vi "get supported types.vi"(8 "error in":errorcluster, 11 "EthernetIP configuration in":refnum<class "EIP Tags Configuration.lvclass">) -> (0 "error out":errorcluster, 2 "supported types":T1[](array[typedef]), 3 "EthernetIP configuration out":refnum<class "EIP Tags Configuration.lvclass">)   [LabVIEW 2013, in "EIP Tags Configuration.lvclass"]
doc: "Provides an interface for determining the targets supported by a given configuration/runtime class pairing. This should be overridden by any useful child class."
uses:
  EIP Tags Configuration.lvclass
  <vilib>/NI/Tag Bus/tag/Data Type.ctl
  <vilib>/NI/Tag Bus/tag/tag descriptor.lvclass
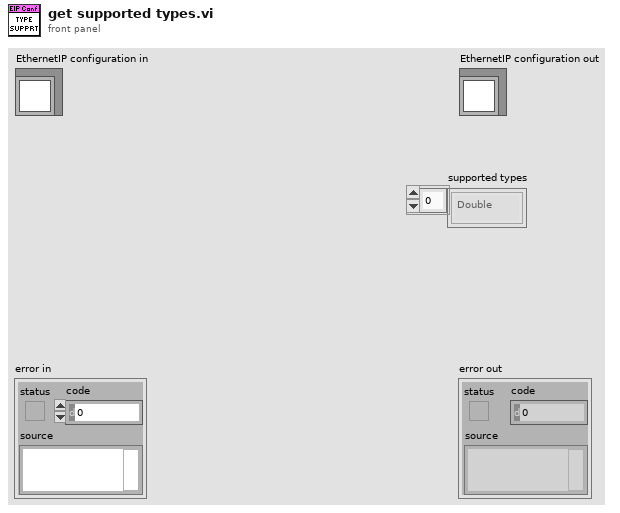
[diagram p1: front panel]
types:
  T1 = typedef "tag bus.lvlib/tag descriptor.lvclass/Data Type.ctl" = enum16{"Double", "Single", "I64", "I32", "I16", "I8", "U64", "U32", "U16", "U8", "Boolean", "String", "Array of Double", "Array of Single", "Array of I64", "Array of I32", "Array of I16", "Array of I8", "Array of U64", "Array of U32", "Array of U16", "Array of U8", "Array of Boolean", "Array of String"}
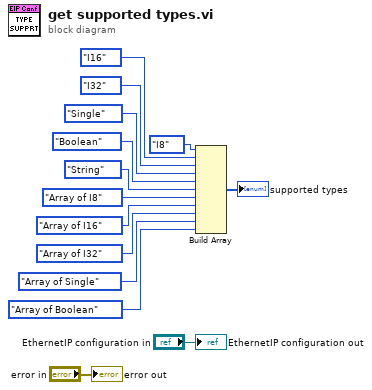
[diagram p0: block diagram]
diagram:
  n1 = Build Array(Data_Type."I8" ("Data Type"), Data_Type."I16" ("Data Type"), Data_Type."I32" ("Data Type"), Data_Type."Single" ("Data Type"), Data_Type."Boolean" ("Data Type"), Data_Type."String" ("Data Type"), Data_Type."Array of I8" ("Data Type"), Data_Type."Array of I16" ("Data Type"), Data_Type."Array of I32" ("Data Type"), Data_Type."Array of Single" ("Data Type"), Data_Type."Array of Boolean" ("Data Type")) -> (→"supported types":T1[])
  "error out" <- "error in"
  "EthernetIP configuration out" <- "EthernetIP configuration in"
